vi "Write Configurations V1.00.vi"(0 "CCD Scan Parameters.Data path":path, 1 "FieldRamp Parameters":dbl[][](array[numeric])=[[0.0, 30.0, 1.0, 400.0], [30.0, 0.0, -1.0, 400.0], [0.0, -30.0, -1.0, 400.0], [-30.0, 0.0, 1.0, 400.0], [0.0, 30.0, 0.5, 200.0], [30.0, 0.0, -0.5, 200.0]] step=1.0 format="%.2f", 2 "Control Parameters":T1={"Grating Density"=enum."1800", "Offset"=0.0, "Save All Data in ONE file"=FALSE, "Auto Save Data"=FALSE, "Most recent saved file"=path "", "Filename Prefix"="MyData", "Extension"=4, "Suffix"="", "Current Path"=path "/DATA"} {"Extension" items=["DOS field", "\".001\",\".002\", ...", "001 (No dot)", "\".A\",\".B\", ...", "±Field", "pField nField", "Temperature", "User Defined"]; "Offset" format="%.2f"}, 3 "CCD Scan Parameters.INI path":path, 5 "SaveParameters(T)/DataBuffer(F)?":bool, 6 "Parameters#2":T3={"MaxBufferSize"=2, "Mag GPIB Address"=5, "Max Current (kA)"=36.0, "LTC-GPIB Address"="", "Temp Tolerance"=1.0} {"Temp Tolerance" format="%.2f"; "Max Current (kA)" format="%.2f"}, 7 "X-Axis Array":dbl[][](array[numeric])=array1025x10[10250 elements] format="%.2f", 8 "Background":i32[](array[numeric])=[1198, 1190, 1193, 1194, 1189, 1188, 1196, 1190, 1202, 1191, 1193, 1192, 1199, 1189, 1194, 1189, 1197, 1191, 1187, 1192, 1195, 1189, 1195, 1191, 1199, 1194, 1192, 1191, 1193, 1197, 1193, 1193, 1194, 1200, 1191, 1190, 1187, 1195, 1189, 1188, 1191, 1194, 1187, 1192, 1198, 1193, 1190, 1192, 1190, 1193, 1191, 1190, 1191, 1189, 1192, 1194, 1190, 1193, 1193, 1191, 1194, 1182, 1190, 1188, 1199, 1192, 1196, 1195, 1186, 1189, 1188, 1185, 1194, 1187, 1193, 1194, 1190, 1189, 1189, 1187, 1196, 1195, 1191, 1197, 1192, 1200, 1187, 1194, 1189, 1193, 1195, 1196, 1186, 1192, 1190, 1194, 1194, 1190, 1191, 1193, 1197, 1197, 1185, 1199, 1190, 1195, 1196, 1184, 1193, 1193, 1193, 1191, 1189, 1190, 1199, 1193, 1191, 1194, 1191, 1192, 1186, 1190, 1194, 1189, 1194, 1190, 1191, 1192, 1192, 1196, 1192, 1192, 1189, 1193, 1198, 1186, 1191, 1193, 1187, 1194, 1190, 1190, 1191, 1189, 1194, 1195, 1189, 1192, 1185, 1193, 1192, 1192, 1189, 1191, 1191, 1190, 1196, 1194, 1193, 1191, 1189, 1191, 1196, 1192, 1192, 1189, 1196, 1191, 1193, 1192, 1188, 1190, 1194, 1192, 1185, 1191, 1194, 1191, 1189, 1195, 1192, 1196, 1190, 1193, 1191, 1189, 1194, 1195, 1191, 1187, 1190, 1196, 1196, 1192, 1197, 1191, 1189, 1192, 1192, 1200, 1192, 1193, 1190, 1192, 1187, 1198, 1186, 1196, 1201, 1199, 1200, 1191, 1196, 1200, 1192, 1191, 1193, 1185, 1192, 1194, 1186, 1190, 1188, 1189, 1201, 1197, 1191, 1194, 1193, 1194, 1195, 1198, 1200, 1192, 1192, 1193, 1193, 1195, 1187, 1193, 1192, 1187, 1189, 1186, 1191, 1197, 1191, 1200, 1194, 1192, 1187, 1196, 1191, 1191, 1196, 1187, 1190, 1193, 1189, 1193, 1190, 1188, 1188, 1190, 1197, 1188, 1191, 1195, 1188, 1191, 1188, 1194, 1193, 1187, 1200, 1192, 1197, 1190, 1196, 1200, 1191, 1189, 1193, 1189, 1186, 1196, 1185, 1198, 1195, 1186, 1191, 1197, 1191, 1193, 1195, 1193, 1191, 1198, 1189, 1183, 1200, 1197, 1192, 1192, 1192, 1196, 1191, 1190, 1194, 1188, 1198, 1193, 1195, 1190, 1187, 1192, 1191, 1195, 1188, 1190, 1191, 1187, 1189, 1185, 1189, 1196, 1198, 1191, 1190, 1196, 1197, 1193, 1187, 1186, 1195, 1191, 1193, 1192, 1196, 1190, 1192, 1192, 1192, 1190, 1195, 1192, 1191, 1193, 1197, 1184, 1190, 1188, 1192, 1194, 1190, 1193, 1195, 1195, 1194, 1189, 1193, 1191, 1194, 1186, 1189, 1192, 1191, 1182, 1190, 1197, 1194, 1188, 1193, 1191, 1186, 1194, 1197, 1193, 1191, 1187, 1194, 1194, 1191, 1189, 1195, 1194, 1189, 1196, 1187, 1186, 1192, 1194, 1196, 1191, 1193, 1191, 1188, 1190, 1199, 1198, 1196, 1196, 1190, 1194, 1191, 1194, 1187, 1195, 1190, 1194, 1196, 1194, 1189, 1193, 1189, 1194, 1189, 1195, 1192, 1194, 1193, 1191, 1197, 1187, 1189, 1189, 1188, 1197, 1192, 1189, 1193, 1194, 1183, 1202, 1187, 1192, 1184, 1188, 1186, 1193, 1189, 1195, 1189, 1193, 1197, 1189, 1194, 1191, 1194, 1192, 1191, 1191, 1196, 1194, 1190, 1193, 1192, 1195, 1197, 1198, 1193, 1202, 1196, 1194, 1194, 1190, 1193, 1190, 1195, 1192, 1187, 1194, 1197, 1190, 1194, 1189, 1198, 1192, 1191, 1192, 1192, 1191, 1191, 1193, 1191, 1191, 1198, 1186, 1192, 1185, 1185, 1188, 1194, 1196, 1194, 1195, 1190, 1194, 1191, 1190, 1195, 1191, 1191, 1195, 1192, 1194, 1201, 1187, 1191, 1195, 1187, 1192, 1192, 1193, 1200, 1188, 1189, 1189, 1197, 1189, 1188, 1197, 1195, 1191, 1189, 1190, 1195, 1189, 1191, 1194, 1186, 1192, 1190, 1191, 1188, 1195, 1192, 1191, 1191, 1199, 1190, 1190, 1190, 1192, 1187, 1193, 1197, 1197, 1186, 1193, 1189, 1192, 1197, 1184, 1187, 1188, 1192, 1192, 1192, 1189, 1192, 1190, 1194, 1191, 1186, 1196, 1194, 1189, 1193, 1191, 1186, 1189, 1193, 1195, 1196, 1197, 1199, 1194, 1190, 1193, 1194, 1190, 1198, 1196, 1194, 1195, 1194, 1184, 1188, 1195, 1197, 1190, 1194, 1190, 1191, 1195, 1198, 1188, 1193, 1194, 1195, 1198, 1195, 1191, 1197, 1192, 1198, 1190, 1196, 1191, 1194, 1188, 1189, 1198, 1192, 1198, 1195, 1185, 1191, 1193, 1192, 1197, 1195, 1195, 1195, 1193, 1190, 1190, 1190, 1198, 1195, 1191, 1194, 1190, 1190, 1194, 1194, 1195, 1192, 1190, 1194, 1195, 1192, 1192, 1194, 1189, 1192, 1193, 1188, 1194, 1195, 1196, 1193, 1192, 1201, 1191, 1198, 1197, 1191, 1192, 1191, 1194, 1193, 1188, 1192, 1189, 1183, 1189, 1190, 1192, 1189, 1196, 1193, 1197, 1185, 1193, 1189, 1191, 1196, 1195, 1193, 1193, 1191, 1189, 1193, 1192, 1192, 1192, 1190, 1191, 1193, 1193, 1197, 1195, 1189, 1193, 1188, 1194, 1197, 1194, 1195, 1196, 1190, 1194, 1188, 1197, 1195, 1191, 1195, 1192, 1194, 1188, 1190, 1197, 1197, 1191, 1187, 1197, 1191, 1193, 1188, 1191, 1194, 1193, 1195, 1192, 1195, 1189, 1193, 1193, 1195, 1190, 1192, 1196, 1188, 1187, 1193, 1192, 1192, 1194, 1185, 1199, 1190, 1193, 1191, 1198, 1189, 1190, 1191, 1190, 1193, 1195, 1186, 1190, 1193, 1191, 1189, 1197, 1193, 1198, 1190, 1192, 1193, 1191, 1196, 1193, 1196, 1190, 1190, 1198, 1192, 1199, 1198, 1190, 1191, 1191, 1196, 1190, 1196, 1195, 1191, 1196, 1195, 1193, 1190, 1190, 1195, 1193, 1187, 1197, 1185, 1191, 1189, 1191, 1193, 1192, 1188, 1196, 1193, 1191, 1193, 1193, 1190, 1192, 1192, 1192, 1195, 1191, 1195, 1189, 1189, 1191, 1191, 1185, 1192, 1191, 1193, 1201, 1199, 1197, 1206, 1201, 1207, 1200, 1198, 1195, 1188, 1194, 1186, 1190, 1197, 1188, 1193, 1196, 1193, 1192, 1192, 1188, 1196, 1186, 1193, 1194, 1188, 1190, 1190, 1192, 1190, 1191, 1191, 1200, 1192, 1199, 1193, 1190, 1190, 1199, 1187, 1193, 1190, 1188, 1194, 1194, 1196, 1194, 1195, 1190, 1187, 1187, 1196, 1193, 1199, 1190, 1193, 1193, 1191, 1198, 1192, 1193, 1192, 1193, 1189, 1189, 1197, 1189, 1194, 1193, 1192, 1185, 1198, 1193, 1189, 1192, 1193, 1196, 1190, 1195, 1189, 1196, 1198, 1190, 1191, 1193, 1186, 1189, 1195, 1188, 1197, 1188, 1191, 1185, 1190, 1193, 1188, 1198, 1192, 1193, 1194, 1194, 1189, 1184, 1193, 1199, 1193, 1192, 1193, 1190, 1196, 1191, 1192, 1189, 1194, 1188, 1189, 1190, 1190, 1192, 1195, 1188, 1190, 1192, 1189, 1197, 1192, 1194, 1187, 1196, 1192, 1194, 1185, 1187, 1187, 1191, 1195, 1190, 1186, 1183, 1194, 1194, 1192, 1192, 1188, 1193, 1195, 1189, 1190, 1191, 1192, 1196, 1186, 1195, 1191, 1185, 1191, 1187, 1190, 1188, 1189, 1187, 1196, 1191, 1190, 1191, 1190, 1196, 1195, 1186, 1187, 1187, 1188, 1194, 1192, 1192, 1192, 1189, 1192, 1191, 1188, 1188, 1187, 1187, 1190, 1186, 1191, 1195, 1192, 1196, 1193, 1192, 1191, 1189, 1187, 1193, 1188, 1189, 1194, 1191, 1185, 1193, 1191, 1196, 1196, 1199, 1195, 1211], 9 "Data Array":dbl[][](array[numeric])=array1025x10[10250 elements] format="%.2f", 10 "Parameters":T2={"Magnetic Field"=0.0, "Temperature"=0.0, "Exposure Time"=0.2, "Mag ID string"="Cell 12", "User Name"="Xing Wei", "Comments"="", "SaveComments?"=1, "X-Axis Unit"=1, "Delimiter"=0, "File Format"=0, "Sample Name"="Ruby"} {"File Format" items=["Macintosh (EOL: CR)", "Unix (EOL: LF)", "DOS/Windows (EOL: CR+LF)"]; "Delimiter" items=["TAB", "COMMA", "SPACE"]; "X-Axis Unit" items=["Point #", "nm", "eV", "meV", "cm-1"]; "SaveComments?" items=["Bare data only", "Saved in the Header Area", "Saved as a Parameter File"]; "Exposure Time" format="%.2f"; "Temperature" format="%.2f"; "Magnetic Field" format="%.2f"}) -> (4 "Done":bool)   [LabVIEW 2024]
uses:
  Parameters#2.ctl
  Parameters#1.ctl
  Parameters_Control.ctl
  <vilib>/Utility/config.llb/Write Key (String).vi
  <vilib>/Utility/config.llb/Write Key (U32).vi
  <vilib>/Utility/config.llb/Write Key (I32).vi
  <vilib>/Utility/config.llb/Write Key (Double).vi
  <vilib>/Utility/config.llb/Write Key (Boolean).vi
  <vilib>/Utility/config.llb/Write Key (Path).vi
  <vilib>/Utility/config.llb/NI_LVConfig.lvlib
panel:
  out "FieldRampSize":i32[](array[numeric])=[6, 4]
  out "X-size":i32[](array[numeric])=[1025, 10]
  out "Y-size":i32[](array[numeric])=[1025, 10]
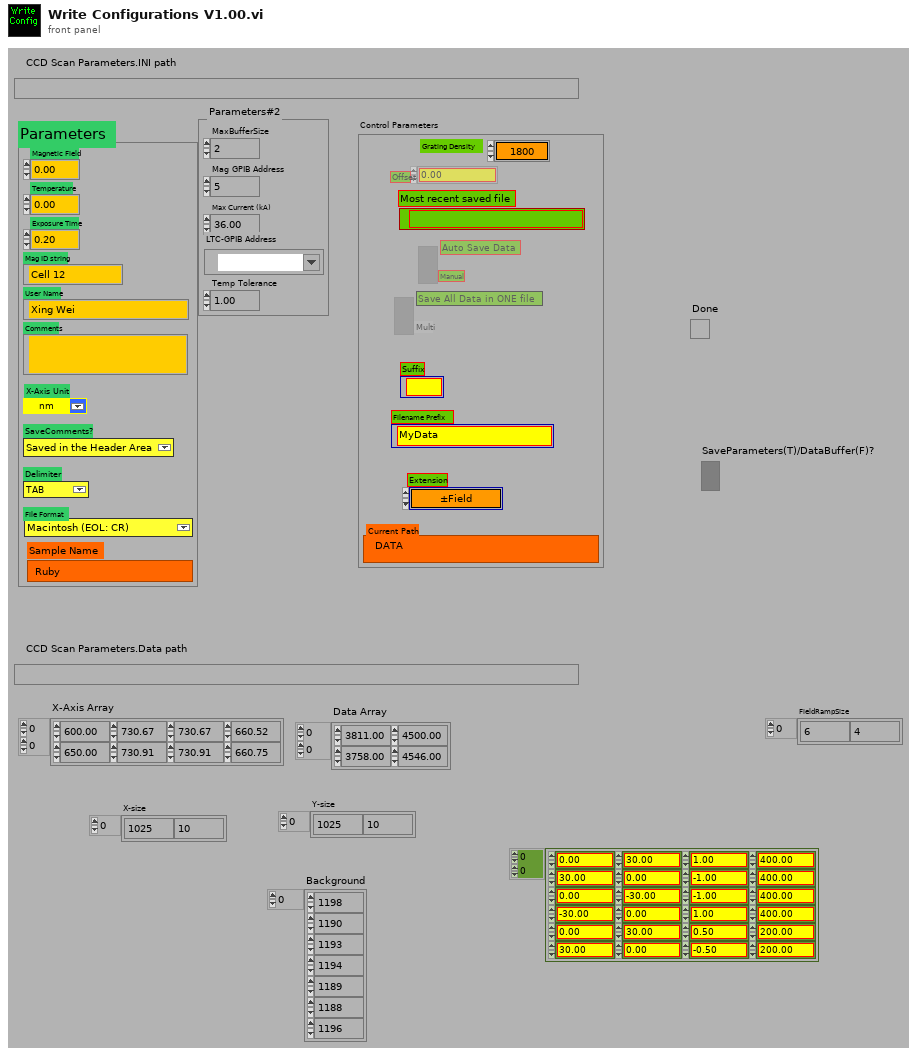
[diagram p1: front panel]
types:
  T1 = typedef "Parameters_Control.ctl" = cluster{"Grating Density":enum16{"150", "300", "600", "1200", "1800"}, "Offset":dbl, "Save All Data in ONE file":bool, "Auto Save Data":bool, "Most recent saved file":path, "Filename Prefix":string, "Extension":u16, "Suffix":string, "Current Path":path}
  T2 = typedef "Parameters#1.ctl" = cluster{"Magnetic Field":dbl, "Temperature":dbl, "Exposure Time":dbl, "Mag ID string":string, "User Name":string, "Comments":string, "SaveComments?":u16, "X-Axis Unit":u16, "Delimiter":u16, "File Format":u16, "Sample Name":string}
  T3 = typedef "Parameters#2.ctl" = cluster{"MaxBufferSize":i32, "Mag GPIB Address":i32, "Max Current (kA)":dbl, "LTC-GPIB Address":refnum<visa-resource-name>, "Temp Tolerance":dbl}
  T4 = enum16{"open", "open or create", "create or replace", "create"}
  T5 = typedef "NI_LVConfig.lvlib/Config Data RefNum.ctl" = refnum<k1>
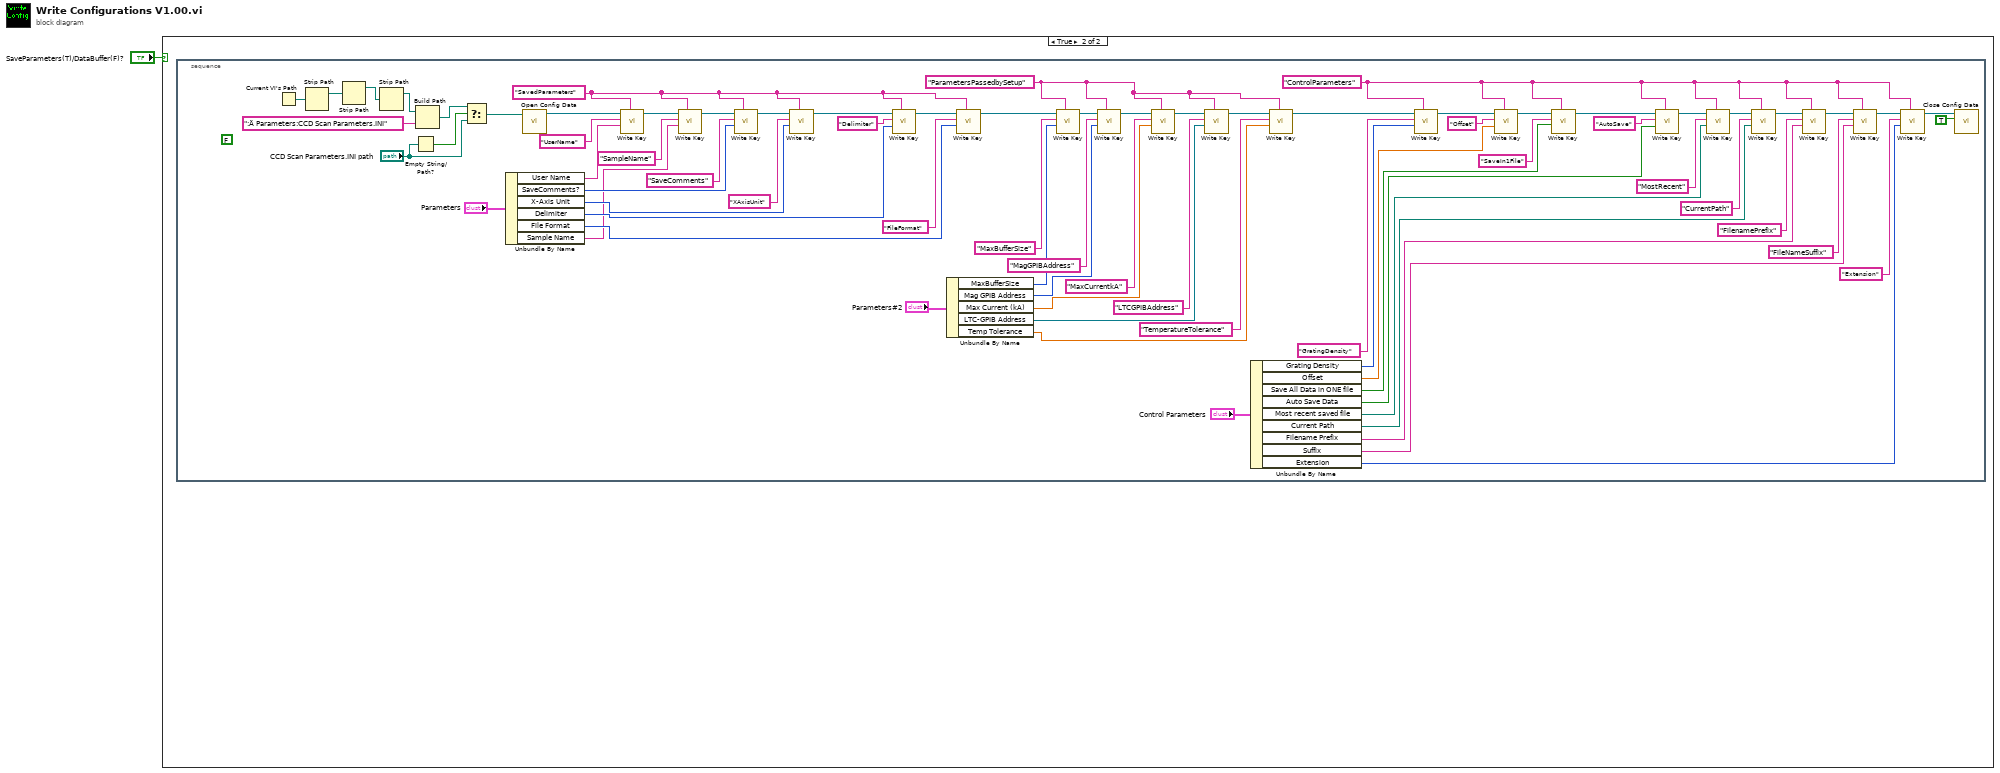
[diagram p0: block diagram]
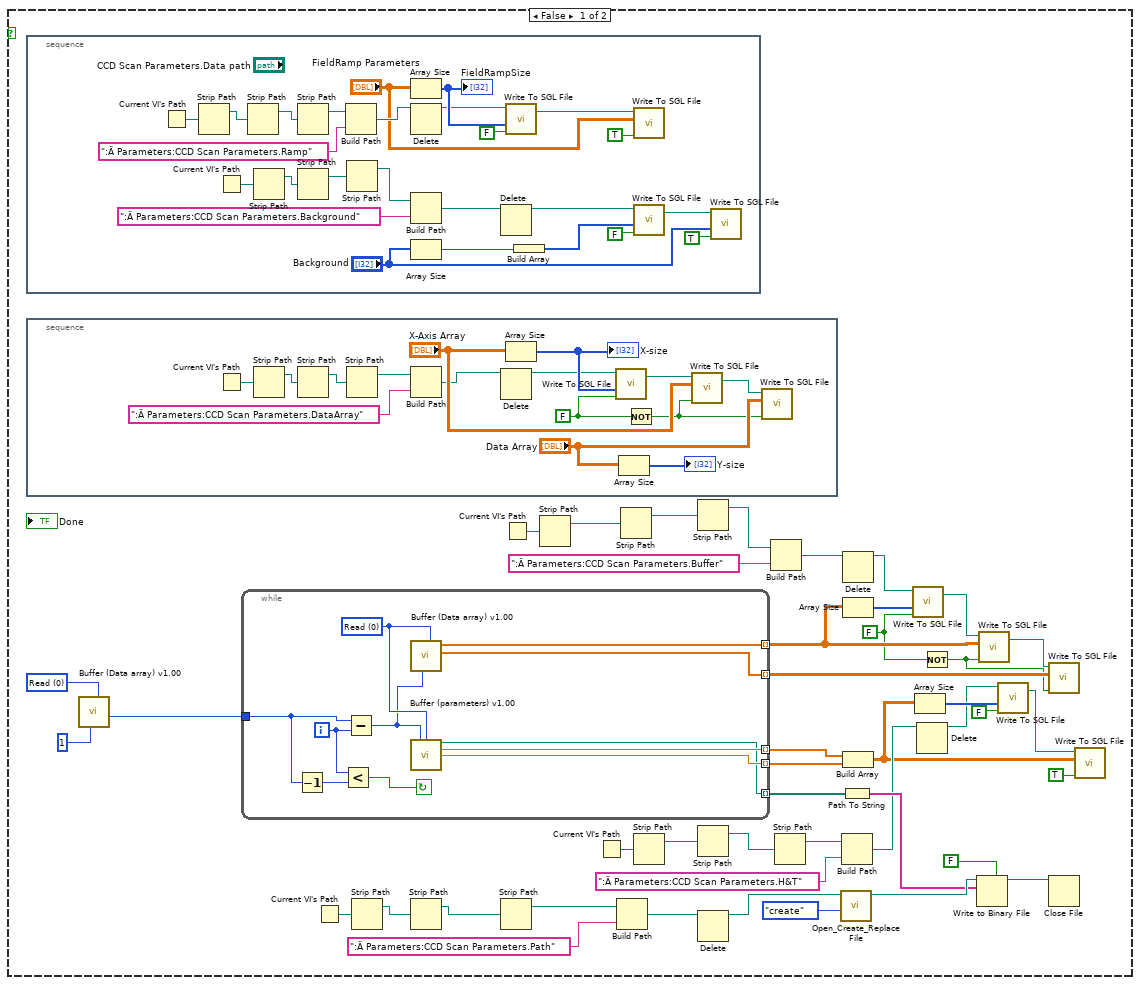
[diagram p2: hidden frame]
diagram:
  n1 = case shown="True" "SaveParameters(T)/DataBuffer(F)?" {
    frame False {
      w20 = FALSE ("append to file? (new file:F)")
      w45 = u16 0 items=["Read", "Write", "Initialize"] ("Read(0) or Write(1)")
      n2 = stacked-sequence {
        frame #0 {
          n3 = Current VI's Path() -> (path=w71:path)
          n4 = Strip Path(path=w71) -> (stripped path=w75:path)  [unwired: 1 out]
          n5 = Current VI's Path() -> (path=w62:path)
          n6 = Strip Path(path=w75) -> (stripped path=w74:path)  [unwired: 1 out]
          n7 = Strip Path(path=w62) -> (stripped path=w66:path)  [unwired: 1 out]
          n8 = Strip Path(path=w74) -> (stripped path=w72:path)  [unwired: 1 out]
          n9 = Strip Path(path=w66) -> (stripped path=w65:path)  [unwired: 1 out]
          n10 = Build Path(base path=w72, name or relative path=":Ä Parameters:CCD Scan Parameters.Ramp") -> (appended path=w69:path)
          n11 = Strip Path(path=w65) -> (stripped path=w63:path)  [unwired: 1 out]
          n12 = Array Size(array="FieldRamp Parameters") -> (size(s)=w80:i32[])
          "FieldRampSize" <- w80
          n13 = Delete(path (use dialog)=w69) -> (deleted path=w70:path)  [unwired: 4 in, 2 out]
          n14 = Build Path(base path=w63, name or relative path=":Ä Parameters:CCD Scan Parameters.Background") -> (appended path=w61:path)
          n15 = Array Size(array="Background") -> (size(s)=w79:i32)
          n16 = Delete(path (use dialog)=w61) -> (deleted path=w60:path)  [unwired: 4 in, 2 out]
          n17 = call <vilib>:"Write To SGL File.vi"("append to file? (new file:F)"=FALSE, "1D array"=w80, "file path (dialog if empty)"=w70) -> ("new file path (Not A Path if cancelled)"=w81:path)  [unwired: 4 in]
          n18 = Build Array(w79) -> (w78:i32[])
          n19 = call <vilib>:"Write To SGL File.vi"("append to file? (new file:F)"=TRUE, "2D array"="FieldRamp Parameters", "file path (dialog if empty)"=w81) -> ()  [unwired: 4 in, 1 out]
          n20 = call <vilib>:"Write To SGL File.vi"("append to file? (new file:F)"=FALSE, "1D array"=w78, "file path (dialog if empty)"=w60) -> ("new file path (Not A Path if cancelled)"=w77:path)  [unwired: 4 in]
          n21 = call <vilib>:"Write To SGL File.vi"("append to file? (new file:F)"=TRUE, "1D array"="Background", "file path (dialog if empty)"=w77) -> ()  [unwired: 4 in, 1 out]
        }
      }
      n22 = stacked-sequence {
        frame #0 {
          w85 = FALSE ("append to file? (new file:F)")
          n23 = Current VI's Path() -> (path=w91:path)
          n24 = Strip Path(path=w91) -> (stripped path=w95:path)  [unwired: 1 out]
          n25 = Strip Path(path=w95) -> (stripped path=w94:path)  [unwired: 1 out]
          n26 = Strip Path(path=w94) -> (stripped path=w92:path)  [unwired: 1 out]
          n27 = Build Path(base path=w92, name or relative path=":Ä Parameters:CCD Scan Parameters.DataArray") -> (appended path=w82:path)
          n28 = Delete(path (use dialog)=w82) -> (deleted path=w84:path)  [unwired: 4 in, 2 out]
          n29 = Array Size(array="X-Axis Array") -> (size(s)=w87:i32[])
          "X-size" <- w87
          n30 = call <vilib>:"Write To SGL File.vi"("append to file? (new file:F)"=w85, "1D array"=w87, "file path (dialog if empty)"=w84) -> ("new file path (Not A Path if cancelled)"=w86:path)  [unwired: 4 in]
          n31 = Array Size(array="Data Array") -> (size(s)=→"Y-size":i32[])
          n32 = Not(x=w85) -> (.not. x?=w83:bool)
          n33 = call <vilib>:"Write To SGL File.vi"("append to file? (new file:F)"=w83, "2D array"="X-Axis Array", "file path (dialog if empty)"=w86) -> ("new file path (Not A Path if cancelled)"=w89:path)  [unwired: 4 in]
          n34 = call <vilib>:"Write To SGL File.vi"("append to file? (new file:F)"=w83, "2D array"="Data Array", "file path (dialog if empty)"=w89) -> ()  [unwired: 4 in, 1 out]
        }
      }
      n35 = call "Buffer (Data array) v1.00.vi"("Action"=w45, "Read#"=1 ("Buffer Size or Read#")) -> ("Current Buffer Size"=w43:i32)  [unwired: 6 in, 3 out]
      n36 = while {
        tunnel: [w48] -> w29 mode=indexing
        tunnel: [w49] -> w10 mode=indexing
        tunnel: [w50] -> w4 mode=indexing
        tunnel: [w53] -> w38 mode=indexing
        tunnel: [w54] -> w39 mode=indexing
        tunnel: w43 -> [w47]
        i -> [w56]
        stop <- w55 continue-if-true
        w52 = u16 0 items=["Read", "Write", "Initialize"] ("Read(0) or Write(1)")
        n37 = Decrement(x=w47) -> (x-1=w46:i32)
        n38 = Less?(x=w56, y=w46) -> (x < y?=w55:bool)
        n39 = Subtract(x=w47, y=w56) -> (x-y=w51:i32)
        n40 = call "Buffer (Data array) v1.00.vi"("Action"=w52, "Read#"=w51) -> ("Y-Data out"=w53:dbl[], "X-Data out"=w54:dbl[])  [unwired: 6 in, 2 out]
        n41 = call "Buffer (parameters) v1.00.vi"("Read#"=w51, "Action"=w52) -> ("FilePath out"=w48:path, "Field Out"=w50:dbl, "Temperature Out"=w49:dbl)  [unwired: 9 in, 2 out]
      }
      n42 = Current VI's Path() -> (path=w33:path)
      n43 = Strip Path(path=w33) -> (stripped path=w37:path)  [unwired: 1 out]
      n44 = Strip Path(path=w37) -> (stripped path=w36:path)  [unwired: 1 out]
      n45 = Strip Path(path=w36) -> (stripped path=w34:path)  [unwired: 1 out]
      n46 = Current VI's Path() -> (path=w23:path)
      n47 = Strip Path(path=w23) -> (stripped path=w27:path)  [unwired: 1 out]
      n48 = Current VI's Path() -> (path=w12:path)
      n49 = Build Path(base path=w34, name or relative path=":Ä Parameters:CCD Scan Parameters.Path") -> (appended path=w19:path)
      n50 = Strip Path(path=w27) -> (stripped path=w26:path)  [unwired: 1 out]
      n51 = Strip Path(path=w12) -> (stripped path=w16:path)  [unwired: 1 out]
      n52 = Strip Path(path=w26) -> (stripped path=w24:path)  [unwired: 1 out]
      n53 = Strip Path(path=w16) -> (stripped path=w15:path)  [unwired: 1 out]
      n54 = Delete(path (use dialog)=w19) -> (deleted path=w18:path)  [unwired: 4 in, 2 out]
      n55 = Build Path(base path=w24, name or relative path=":Ä Parameters:CCD Scan Parameters.Buffer") -> (appended path=w22:path)
      n56 = Strip Path(path=w15) -> (stripped path=w13:path)  [unwired: 1 out]
      n57 = call <vilib>:"Open_Create_Replace File.vi"("function (open:0)"=T4."create", "file path"=w18) -> ("refnum"=w31:refnum<file>)  [unwired: 6 in, 3 out]
      n58 = Path To String(path=w29) -> (string=w28:string[])
      n59 = Build Path(base path=w13, name or relative path=":Ä Parameters:CCD Scan Parameters.H&T") -> (appended path=w11:path)
      n60 = Delete(path (use dialog)=w22) -> (deleted path=w21:path)  [unwired: 4 in, 2 out]
      n61 = Array Size(array=w39) -> (size(s)=w42:i32[])
      n62 = Build Array(w4, w10) -> (w3:dbl[][])
      n63 = call <vilib>:"Write To SGL File.vi"("append to file? (new file:F)"=w20, "1D array"=w42, "file path (dialog if empty)"=w21) -> ("new file path (Not A Path if cancelled)"=w41:path)  [unwired: 4 in]
      n64 = Array Size(array=w3) -> (size(s)=w9:i32[])
      n65 = Delete(path (use dialog)=w11) -> (deleted path=w8:path)  [unwired: 4 in, 2 out]
      n66 = Not(x=w20) -> (.not. x?=w17:bool)
      n67 = Write to Binary File(file (use dialog)=w31, data=w28, 5:FALSE ("prepend array or string size? (T)")) -> (refnum out=w30:refnum<file>)  [unwired: 3 in, 2 out]
      n68 = call <vilib>:"Write To SGL File.vi"("append to file? (new file:F)"=w17, "2D array"=w39, "file path (dialog if empty)"=w41) -> ("new file path (Not A Path if cancelled)"=w40:path)  [unwired: 4 in]
      n69 = call <vilib>:"Write To SGL File.vi"("append to file? (new file:F)"=FALSE, "1D array"=w9, "file path (dialog if empty)"=w8) -> ("new file path (Not A Path if cancelled)"=w7:path)  [unwired: 4 in]
      n70 = call <vilib>:"Write To SGL File.vi"("append to file? (new file:F)"=w17, "2D array"=w38, "file path (dialog if empty)"=w40) -> ()  [unwired: 4 in, 1 out]
      n71 = Close File(refnum=w30) -> ()  [unwired: 1 in, 2 out]
      n72 = call <vilib>:"Write To SGL File.vi"("append to file? (new file:F)"=TRUE, "2D array"=w3, "file path (dialog if empty)"=w7) -> ()  [unwired: 4 in, 1 out]
    }
    frame True {
      n73 = stacked-sequence {
        frame #0 {
          (unwired) FALSE ("write configuration file? (T)")
          w97 = "ControlParameters" ("section")
          w128 = "ParametersPassedbySetup" ("section")
          w144 = "SavedParameters" ("section")
          n74 = Current VI's Path() -> (path=w167:path)
          n75 = Strip Path(path=w167) -> (stripped path=w172:path)  [unwired: 1 out]
          n76 = Strip Path(path=w172) -> (stripped path=w171:path)  [unwired: 1 out]
          n77 = Strip Path(path=w171) -> (stripped path=w168:path)  [unwired: 1 out]
          n78 = Empty String/Path?(string/path="CCD Scan Parameters.INI path") -> (empty?=w173:bool)
          n79 = Build Path(base path=w168, name or relative path=":Ä Parameters:CCD Scan Parameters.INI") -> (appended path=w166:path)
          n80 = Select(t=w166, s=w173, f="CCD Scan Parameters.INI path") -> (s? t:f=w162:path)
          n81 = Unbundle By Name("Parameters") -> ("User Name"=w160:string, "SaveComments?"=w158:u16, "X-Axis Unit"=w155:u16, "Delimiter"=w151:u16, "File Format"=w149:u16, "Sample Name"=w145:string)
          n82 = call <vilib>:"Open Config Data.vi"("configuration file path"=w162) -> ("refnum"=w127:T5)  [unwired: 8 in, 2 out]
          n83 = call-poly <vilib>:"Write Key.vi"("section"=w144, "value"=w160, "key"="UserName", "refnum"=w127) -> ("refnum out"=w148:T5)  [unwired: 5 in, 2 out]
          n84 = call-poly <vilib>:"Write Key.vi"("section"=w144, "value"=w145, "key"="SampleName", "refnum"=w148) -> ("refnum out"=w147:T5)  [unwired: 5 in, 2 out]
          n85 = call-poly <vilib>:"Write Key.vi"("section"=w144, "value"=w158, "key"="SaveComments", "refnum"=w147) -> ("refnum out"=w157:T5)  [unwired: 5 in, 2 out]
          n86 = call-poly <vilib>:"Write Key.vi"("section"=w144, "value"=w155, "key"="XAxisUnit", "refnum"=w157) -> ("refnum out"=w154:T5)  [unwired: 5 in, 2 out]
          n87 = call-poly <vilib>:"Write Key.vi"("section"=w144, "value"=w151, "key"="Delimiter", "refnum"=w154) -> ("refnum out"=w153:T5)  [unwired: 5 in, 2 out]
          n88 = Unbundle By Name("Parameters#2") -> ("MaxBufferSize"=w138:i32, "Mag GPIB Address"=w137:i32, "Max Current (kA)"=w136:dbl, "LTC-GPIB Address"=w135:refnum<visa-resource-name>, "Temp Tolerance"=w134:dbl)
          n89 = call-poly <vilib>:"Write Key.vi"("section"=w144, "value"=w149, "key"="FileFormat", "refnum"=w153) -> ("refnum out"=w143:T5)  [unwired: 5 in, 2 out]
          n90 = call-poly <vilib>:"Write Key.vi"("section"=w128, "value"=w138, "key"="MaxBufferSize", "refnum"=w143) -> ("refnum out"=w142:T5)  [unwired: 5 in, 2 out]
          n91 = call-poly <vilib>:"Write Key.vi"("section"=w128, "value"=w137, "key"="MagGPIBAddress", "refnum"=w142) -> ("refnum out"=w141:T5)  [unwired: 5 in, 2 out]
          n92 = call-poly <vilib>:"Write Key.vi"("section"=w128, "value"=w136, "key"="MaxCurrentkA", "refnum"=w141) -> ("refnum out"=w140:T5)  [unwired: 5 in, 2 out]
          n93 = call-poly <vilib>:"Write Key.vi"("section"=w128, "value"=w135, "key"="LTCGPIBAddress", "refnum"=w140) -> ("refnum out"=w139:T5)  [unwired: 5 in, 2 out]
          n94 = Unbundle By Name("Control Parameters") -> ("Grating Density"=w115:enum16{"150", "300", "600", "1200", "1800"}, "Offset"=w114:dbl, "Save All Data in ONE file"=w113:bool, "Auto Save Data"=w112:bool, "Most recent saved file"=w111:path, "Current Path"=w110:path, "Filename Prefix"=w109:string, "Suffix"=w108:string, "Extension"=w107:u16)
          n95 = call-poly <vilib>:"Write Key.vi"("section"=w128, "value"=w134, "key"="TemperatureTolerance", "refnum"=w139) -> ("refnum out"=w126:T5)  [unwired: 5 in, 2 out]
          n96 = call-poly <vilib>:"Write Key.vi"("section"=w97, "value"=w115, "key"="GratingDensity", "refnum"=w126) -> ("refnum out"=w125:T5)  [unwired: 5 in, 2 out]
          n97 = call-poly <vilib>:"Write Key.vi"("section"=w97, "value"=w114, "key"="Offset", "refnum"=w125) -> ("refnum out"=w124:T5)  [unwired: 5 in, 2 out]
          n98 = call-poly <vilib>:"Write Key.vi"("section"=w97, "value"=w113, "key"="SaveIn1File", "refnum"=w124) -> ("refnum out"=w123:T5)  [unwired: 5 in, 2 out]
          n99 = call-poly <vilib>:"Write Key.vi"("section"=w97, "value"=w112, "key"="AutoSave", "refnum"=w123) -> ("refnum out"=w122:T5)  [unwired: 5 in, 2 out]
          n100 = call-poly <vilib>:"Write Key.vi"("section"=w97, "value"=w111, "key"="MostRecent", "refnum"=w122) -> ("refnum out"=w121:T5)  [unwired: 5 in, 2 out]
          n101 = call-poly <vilib>:"Write Key.vi"("section"=w97, "value"=w110, "key"="CurrentPath", "refnum"=w121) -> ("refnum out"=w120:T5)  [unwired: 5 in, 2 out]
          n102 = call-poly <vilib>:"Write Key.vi"("section"=w97, "value"=w109, "key"="FilenamePrefix", "refnum"=w120) -> ("refnum out"=w119:T5)  [unwired: 5 in, 2 out]
          n103 = call-poly <vilib>:"Write Key.vi"("section"=w97, "value"=w108, "key"="FileNameSuffix", "refnum"=w119) -> ("refnum out"=w118:T5)  [unwired: 5 in, 2 out]
          n104 = call-poly <vilib>:"Write Key.vi"("section"=w97, "value"=w107, "key"="Extension", "refnum"=w118) -> ("refnum out"=w117:T5)  [unwired: 5 in, 2 out]
          n105 = call <vilib>:"Close Config Data.vi"("write file if changed (T)"=TRUE ("write configuration file? (F)"), "refnum"=w117) -> ()  [unwired: 8 in, 2 out]
        }
      }
    }
  }
